vi "dfd_MA_No Rate Change Filter.vi"(0 "input data":fxp<+/-,32,32>=4.0, 9 "input valid":bool=TRUE) -> (4 "output data":fxp<+/-,32,32>, 10 "output valid":bool, 14 "ready for input":bool)   [LabVIEW 2017]
uses:
  <vilib>/rvi/Memory/Memory_Emulation/nirvimemoryEmulation.vi
  <vilib>/rvi/Memory/Memory_Emulation/nirvimemoryFastEmulation.vi
  <vilib>/rvi/DataTransferAndStorage/Container/Common/niFpgaContainerGetUniqueNameForEmu.vi
  <vilib>/rvi/Memory/Memory_Emulation/niFpgaMemoryEmulationCacheClearOnFirstRun.vi
  <vilib>/rvi/Memory/Memory_Emulation/nirvimemoryEmulationManagerCache_MakeExclusive.vi
  <vilib>/rvi/Memory/Memory_Emulation/niFpgaMemoryEmulationValidateCache.vi
  <vilib>/rvi/Memory/Memory_Emulation/nirvimemoryEmulationManagerCache_InsertValue.vi
  <vilib>/Utility/error.llb/Clear Errors.vi
  <vilib>/rvi/Memory/Memory_Emulation/nirvimemoryEmulationManagerCache_ReleaseExclusive.vi
  <vilib>/rvi/Memory/Memory_Emulation/nirvimemoryEmulationManagerCache_GetValue.vi
  <vilib>/rvi/Emulation/niFpgaEmulationIsFPGAContextNoSignature.vi
  <vilib>/rvi/Emulation/niFpgaSctlEmulationGetInTimedLoop.vi
  <vilib>/rvi/Memory/Memory_Emulation/nirvimemoryEmulationManagerCache_SetValue.vi
  <vilib>/rvi/Emulation/niFpgaSctlEmulationResourceMgr.vi
  <vilib>/rvi/DataTransferAndStorage/Container/Common/niFpgaContainerSetEmuInfo.vi
  <vilib>/rvi/eio/common/nirviEmuReportErrorAndStop.vi
  <vilib>/rvi/FXPMathLib/basic elements/FxpDiscreteDelay/XNode/nifxpmath_DiscreteDelay.xnode
  <vilib>/rvi/FXPMathLib/basic elements/FxpAddSub/XNode/nifxpmath_AddSub.xnode
  <vilib>/rvi/DataTransferAndStorage/Container/XNode/niFpgaContainer.xnode
  <vilib>/rvi/FXPMathLib/FxpMul/XNode/nifxpmath_Multiplier.xnode
  <vilib>/rvi/LocalResourceManager/LocalResourceManager.xnode
  <vilib>/rvi/FXPMathLib/sim/FxpSim.dll
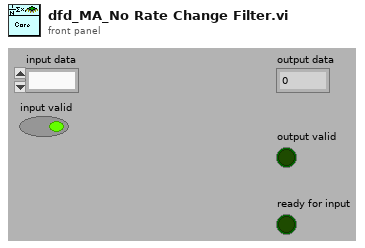
[diagram p1: front panel]
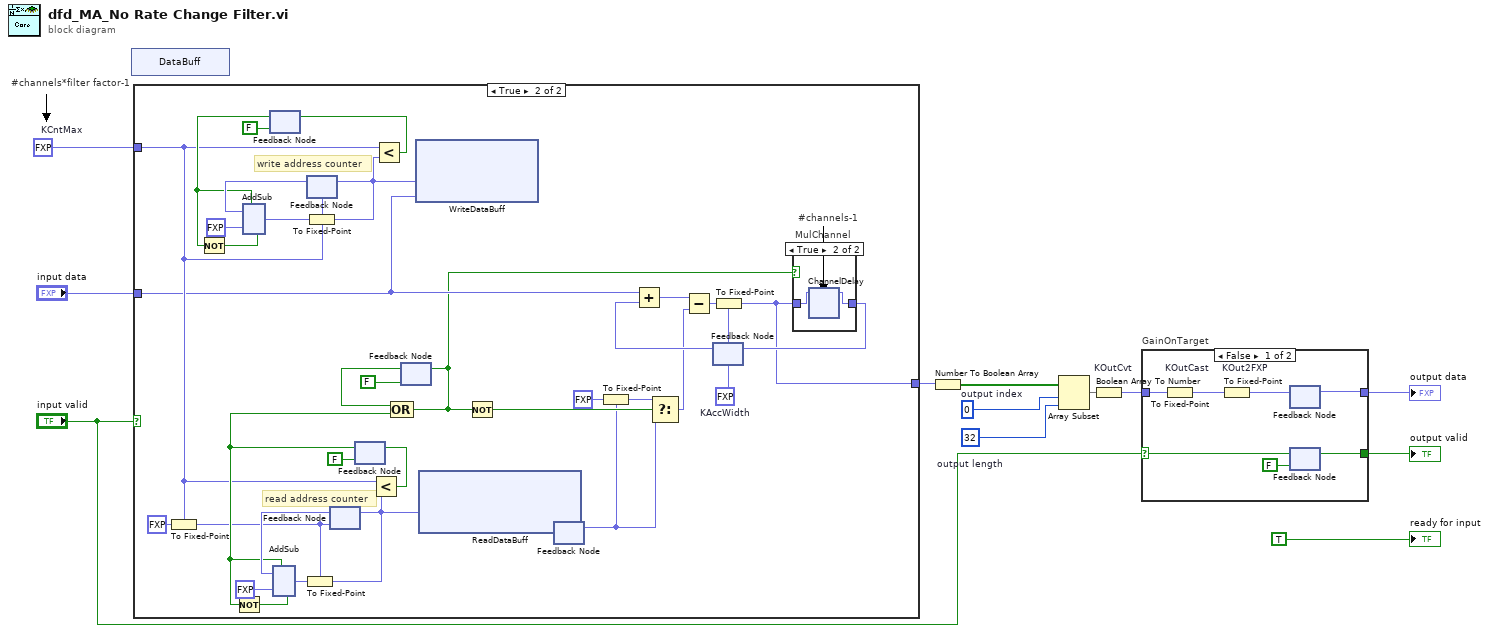
[diagram p0: block diagram]
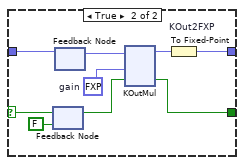
[diagram p2: hidden frame]
diagram:
  w7 = 32  # output length
  w6 = 0  # output index
  w11 = fxp<+,5,5> 1.0  # KCntMax
  # "#channels*filter factor-1"
  n1 = xnode "DataBuff"() -> ()  [unwired: 1 out]
  n2 = case shown="True" "input valid" {
    tunnel: w11 -> [_ w27]
    tunnel: "input data" -> [_ w19]
    tunnel: [_ w14] -> w2
    frame False {
    }
    frame True {
      w20 = fxp<+/-,48,48> 0.0  # KAccWidth
      # "#channels-1"
      # "write address counter"
      # "read address counter"
      n3 = To Fixed-Point(fixed-point type=w27, number=fxp<+,1,1> 0.0 ("y")) -> (fixed-point=w26:fxp<+,5,5>)
      n4 = feedback #1(FALSE) -> (w31:bool)
      n5 = Not(x=w31) -> (.not. x?=w30:bool)
      n6 = feedback #2(w27) -> (w46:fxp<+,5,5>)
      n7 = xnode "AddSub"("x"=w46, "y"=fxp<+,1,1> 0.0, "carry-in"=w30, "use zero instead of x"=w31) -> ("s"=w43:fxp<+,5,5>)  [unwired: 1 out]
      n8 = To Fixed-Point(fixed-point type=w27, number=w43) -> (fixed-point=w40:fxp<+,5,5>)
      n9 = feedback-in #2(w40) -> ()
      n10 = feedback #3(w26) -> (w32:fxp<+,5,5>)
      n11 = feedback #4(FALSE) -> (w29:bool)
      n12 = Not(x=w29) -> (.not. x?=w28:bool)
      n13 = xnode "AddSub"("x"=w32, "y"=fxp<+,1,1> 0.0, "carry-in"=w28, "use zero instead of x"=w29) -> ("s"=w42:fxp<+,5,5>)  [unwired: 1 out]
      n14 = To Fixed-Point(fixed-point type=w26, number=w42) -> (fixed-point=w37:fxp<+,5,5>)
      n15 = feedback-in #3(w37) -> ()
      n16 = Less?(x=w27, y=w37) -> (x < y?=w35:bool)
      n17 = feedback-in #4(w35) -> ()
      n18 = Less?(x=w27, y=w40) -> (x < y?=w39:bool)
      n19 = feedback-in #1(w39) -> ()
      n20 = feedback #5(FALSE) -> (w34:bool)
      n21 = Compound Arithmetic op=OR(w34, w29) -> (w13:bool)
      n22 = feedback-in #5(w13) -> ()
      n23 = xnode "WriteDataBuff"("Address"=w40, "Data"=w19) -> ()  [unwired: 1 in, 1 out]
      n24 = xnode "ReadDataBuff"("Address"=w37) -> ("Data"=w23:fxp<+/-,32,32>)  [unwired: 1 in, 1 out]
      n25 = Not(x=w13) -> (.not. x?=w47:bool)
      n26 = feedback-in #6(w23) -> ()
      n27 = feedback #6() -> (w21:fxp<+/-,32,32>)  [unwired: 1 out]
      n28 = To Fixed-Point(fixed-point type=w21, number=fxp<+/-,32,32> 0.0 ("Data")) -> (fixed-point=w22:fxp<+/-,32,32>)
      n29 = Select(t=w22, s=w47, f=w21) -> (s? t:f=w16:fxp<+/-,32,32>)
      n30 = feedback #7(w20) -> (w18:fxp<+/-,48,48>)
      n31 = Add(x=w19, y=w18) -> (x+y=w17:fxp<+/-,49,49>)
      n32 = Subtract(x=w17, y=w16) -> (x-y=w15:fxp<+/-,49,49>)
      n33 = To Fixed-Point(fixed-point type=w20, number=w15) -> (fixed-point=w14:fxp<+/-,48,48>)
      n34 = case "MulChannel" shown="True" w13 {
        tunnel: w14 -> [w48 w50]
        tunnel: [w48 w49] -> w25
        frame False {
        }
        frame True {
          n35 = xnode ("ChannelDelay")("D"=w50) -> ("Q"=w49:fxp<+/-,48,48>)
        }
      }
      n36 = feedback-in #7(w25) -> ()
    }
  }
  n37 = Number To Boolean Array(number=w2) -> (Boolean array=w9:bool[])
  n38 = Array Subset(array=w9, index=w6, length=w7) -> (w8:bool[])
  n39 = Boolean Array To Number "KOutCvt"(Boolean array=w8) -> (number=w5:fxp<+/-,32,32>)
  n40 = case "GainOnTarget" shown="False" "input valid" {
    selector: "input valid" -> [w185 w194]
    tunnel: [w187 w198] -> w3
    tunnel: [w188 w196] -> w4
    tunnel: w5 -> [w184 w195]
    frame False {
      n41 = To Fixed-Point "KOutCast"(number=w184) -> (fixed-point=w183:fxp<+/-,32,32>)  [unwired: 1 out]
      n42 = To Fixed-Point "KOut2FXP"(number=w183) -> (fixed-point=w186:fxp<+/-,32,32>)  [unwired: 1 out]
      n43 = feedback-in #8(w186) -> ()
      n44 = feedback #8() -> (w188:fxp<+/-,32,32>)  [unwired: 1 out]
      n45 = feedback-in #9(w185) -> ()
      n46 = feedback #9(FALSE ("input valid")) -> (w187:bool)
    }
    frame True {
      w197 = fxp<+/-,16,1> 0.0  # gain
      n47 = feedback-in #10(w194) -> ()
      n48 = feedback #10(FALSE) -> (w192:bool)
      n49 = feedback-in #11(w195) -> ()
      n50 = feedback #11() -> (w193:fxp<+/-,32,32>)  [unwired: 1 out]
      n51 = xnode "KOutMul"("x"=w193, "y"=w197, "input valid"=w192) -> ("x*y"=w190:fxp<+/-,32,32>, "output valid"=w198:bool)  [unwired: 1 in, 1 out]
      n52 = To Fixed-Point "KOut2FXP"(number=w190) -> (fixed-point=w196:fxp<+/-,32,32>)  [unwired: 1 out]
    }
  }
  "output valid" <- w3
  "output data" <- w4
  "ready for input" <- TRUE ("ready for input")
